vi "EnQ.vi"(6 "Priority?":bool, 9 "Msg":refnum<class "Msg.lvclass">, 10 "Msg Q":refnum<data-value>) -> (0 "error out":errorcluster)   [LabVIEW 2021, in "LVCAM.lvlib" / "Msg Q.lvclass"]
uses:
  Msg Q.lvclass
  Msg/Msg.lvclass
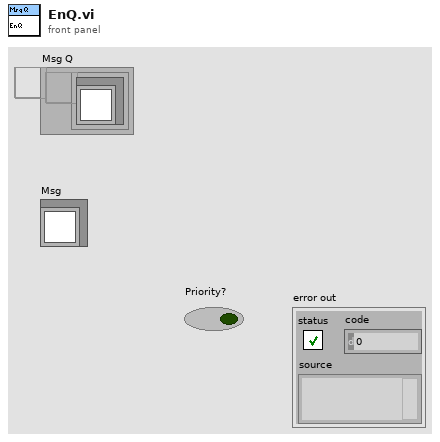
[diagram p1: front panel]
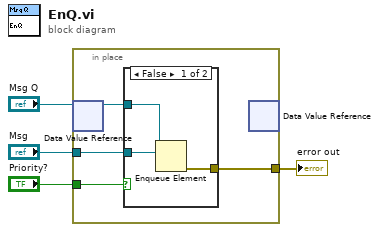
[diagram p0: block diagram]
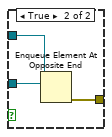
[diagram p2: hidden frame]
diagram:
  n1 = in-place {
    in-place-border: "Msg" -> [w8]
    in-place-border: "Priority?" -> [w7]
    in-place-border: [w6] -> w2
    n2 = in-place-dvr #1("Msg Q") -> (w5:refnum<queue>)  [unwired: 1 out]
    n3 = case shown="False" w7 {
      tunnel: [w11 w12] -> w6
      tunnel: w5 -> [w10 w14]
      tunnel: w8 -> [w9 w13]
      frame False {
        n4 = Enqueue Element(queue=w10, element=w9) -> (error out=w11:errorcluster)  [unwired: 2 in, 2 out]
      }
      frame True {
        n5 = Enqueue Element At Opposite End(queue=w14, element=w13) -> (error out=w12:errorcluster)  [unwired: 2 in, 2 out]
      }
    }
    n6 = in-place-dvr #1() -> ()  [unwired: 1 in, 2 out]
  }
  "error out" <- w2
